vi "Write GIF File (Animated)__ogtk.vi"(6 "delay (ms)":u32[](array[numeric]), 7 "overwrite? (false)":bool, 8 "error in (no error)":errorcluster, 10 "images data":T1[](array[typedef]), 11 "path to GIF file":path) -> (0 "error out":errorcluster, 3 "path":path)   [LabVIEW 2009]
doc: "Writes a multi-frame (animated) Compuserve GIF file. If no path is specified, a file dialog is used to find the file."
uses:
  <vilib>/picture/picture.llb/imagedata.ctl
panel:
  # "Write GIF File (Animated).vi\n\nWrites a multi-frame (animated) Compuserve GIF file. If no path is specified, a file dialog is used to find the file.\n\nPlease visit http://www.OpenG.org to learn about the\nOpen Source LabVIEW software movement.\n\nNOTICE -- YOU MUST LEAVE THIS NOTICE IN PLACE.  PER THE TERMS OF THE LICENSE BELOW, YOU MAY SUBLICENSE THIS SOFTWARE \nIN ANY WAY THAT DOES NOT CONFLICT WITH THIS LICENSE.\n\n### BSD License (http://www.opensource.org/licenses/bsd-license.php) Begin ###\n \nCopyright (c) 2007, Bill Clench <bclench@yahoo.com>\n\nAll rights reserved.\n\nRedistribution and use in source and binary forms, with or without modification, are permitted provided that the following conditions are met:\n\n    * Redistributions of source code must retain the above copyright notice, this list of conditions and the following disclaimer.\n    * Redistributions in binary form must reproduce the above copyright notice, this list of conditions and the following disclaimer in the \n       documentation and/or other materials provided with the distribution.\n    * Neither the name of SciWare, James Kring, Inc., nor the names of its contributors may be used to endorse or promote products derived \n       from this software without specific prior written permission.\n\nTHIS SOFTWARE IS PROVIDED BY THE COPYRIGHT HOLDERS AND CONTRIBUTORS \"AS IS\" AND ANY EXPRESS OR IMPLIED WARRANTIES, \nINCLUDING, BUT NOT LIMITED TO, THE IMPLIED WARRANTIES OF MERCHANTABILITY AND FITNESS FOR A PARTICULAR PURPOSE ARE \nDISCLAIMED. IN NO EVENT SHALL THE COPYRIGHT OWNER OR CONTRIBUTORS BE LIABLE FOR ANY DIRECT, INDIRECT, INCIDENTAL,\n SPECIAL, EXEMPLARY, OR CONSEQUENTIAL DAMAGES (INCLUDING, BUT NOT LIMITED TO, PROCUREMENT OF SUBSTITUTE GOODS OR \nSERVICES; LOSS OF USE, DATA, OR PROFITS; OR BUSINESS INTERRUPTION) HOWEVER CAUSED AND ON ANY THEORY OF LIABILITY, \nWHETHER IN CONTRACT, STRICT LIABILITY, OR TORT (INCLUDING NEGLIGENCE OR OTHERWISE) ARISING IN ANY WAY OUT OF THE USE \nOF THIS SOFTWARE, EVEN IF ADVISED OF THE POSSIBILITY OF SUCH DAMAGE.\n\n### BSD License End ###"
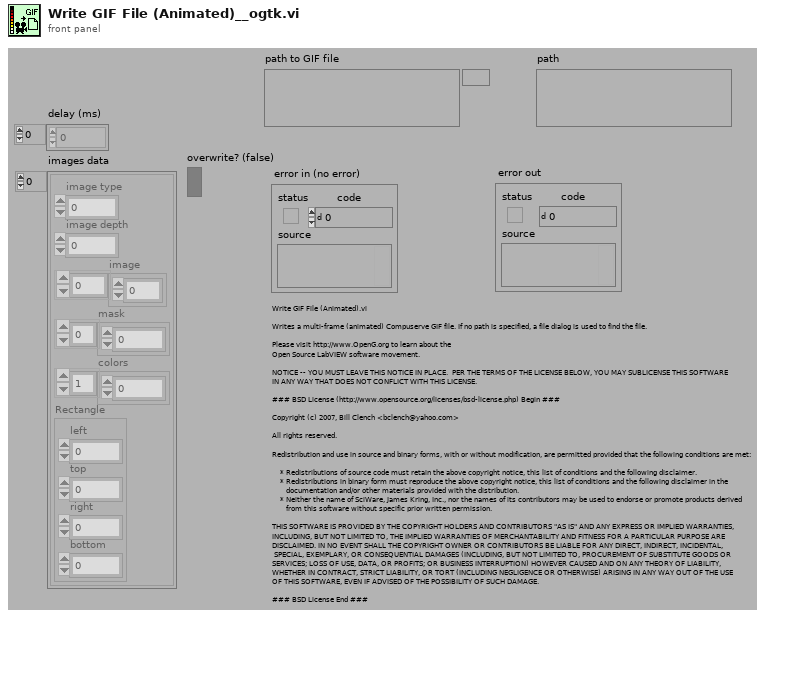
[diagram p1: front panel]
types:
  T1 = typedef "imagedata.ctl" = cluster{"image type":i32, "image depth":i32, "image":u8[], "mask":u8[], "colors":u32[], "Rectangle":cluster{"left":i16, "top":i16, "right":i16, "bottom":i16}}
  T2 = enum32{"existing file", "new file", "new or existing file", "existing dir", "new dir", "new or existing dir", "existing file (use LLBs)", "new file (use LLBs)", "new or existing file (use LLBs)", "new or existing file or directory (use LLBs)", "existing dir (use LLBs)", "new dir (use LLBs)", "new or existing dir (use LLBs)", "existing file or dir", "new file or dir", "new or existing file or dir", "existing file or dir (use LLBs)", "new file or dir (use LLBs)"}
  T3 = enum16{"open", "replace", "create", "open or create", "replace or create", "replace or create with confirmation"}
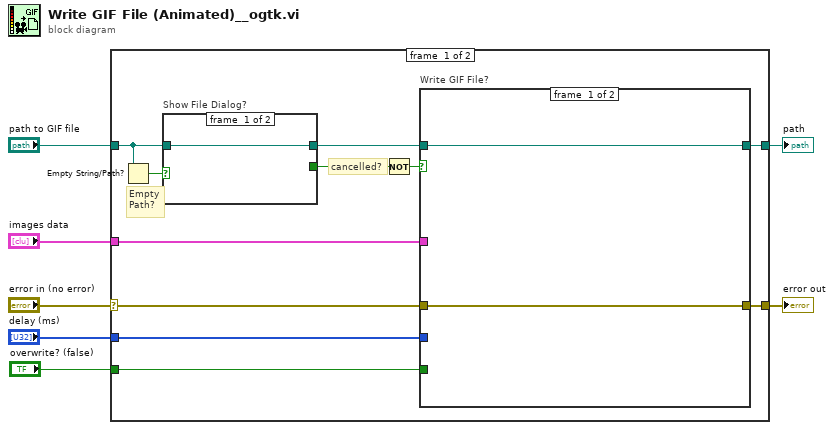
[diagram p0: block diagram]
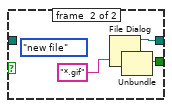
[diagram p2: hidden frame]
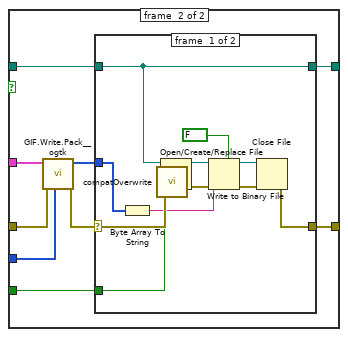
[diagram p3: hidden frame]
diagram:
  n1 = case shown="No Error" "error in (no error)" {
    selector: "error in (no error)" -> [w8 w49]
    tunnel: "images data" -> [w18 _]
    tunnel: [w17 w49] -> w6
    tunnel: "path to GIF file" -> [w15 w50]
    tunnel: "delay (ms)" -> [w12 _]
    tunnel: "overwrite? (false)" -> [w11 _]
    tunnel: [w10 w50] -> w2
    frame #0 {
      # "Empty\nPath?"
      # "cancelled?"
      n2 = Empty String/Path?(string/path=w15) -> (empty?=w16:bool)
      n3 = case "Show File Dialog?" shown="True" w16 {
        tunnel: w15 -> [w19 _]
        tunnel: [w19 w23] -> w13
        tunnel: [_ w21] -> w14
        frame #0 {
        }
        frame #1 {
          (unwired) T2."new file" ("select mode (2)")
          n4 = File Dialog(6:"*.gif") -> (0:w20:errorcluster, 1:w21:bool, 3:w23:path)  [unwired: 6 in, 1 out]
          n5 = Unbundle(w20) -> ()  [unwired: 3 out]
        }
      }
      n6 = Not(x=w14) -> (.not. x?=w9:bool)
      n7 = case "Write GIF File?" shown="True" w9 {
        tunnel: w8 -> [w25 w34]
        tunnel: w18 -> [_ w27]
        tunnel: [w25 w32] -> w17
        tunnel: w13 -> [w24 w30]
        tunnel: w12 -> [_ w29]
        tunnel: w11 -> [_ w28]
        tunnel: [w24 w26] -> w10
        frame #0 {
        }
        frame #1 {
          n8 = call "GIF.Write.Pack__ogtk.vi"("Delay (ms)"=w29, "error in (no error)"=w34, "Images"=w27) -> ("error out"=w33:errorcluster, "Array"=w31:u8[])  [unwired: 7 in]
          n9 = case shown="No Error" w33 {
            selector: w33 -> [w46 w48]
            tunnel: [w45 w48] -> w32
            tunnel: w31 -> [w44 _]
            tunnel: w30 -> [w41 w47]
            tunnel: w28 -> [w42 _]
            tunnel: [w41 w47] -> w26
            frame #0 {
              n10 = Byte Array To String(unsigned byte array=w44) -> (string=w43:string)
              n11 = call <vilib>:"compatOverwrite.vi"("overwrite (F)"=w42) -> ("overwrite?"=w35:T3)
              n12 = Open/Create/Replace File(file path (use dialog)=w41, error in=w46, operation (0:open)=w35) -> (refnum out=w40:refnum<file>, error out=w39:errorcluster)  [unwired: 3 in, 1 out]
              n13 = Write to Binary File(file (use dialog)=w40, data=w43, error in=w39, 5:FALSE ("prepend array or string size? (T)")) -> (refnum out=w38:refnum<file>, error out=w37:errorcluster)  [unwired: 2 in, 1 out]
              n14 = Close File(refnum=w38, error in=w37) -> (error out=w45:errorcluster)  [unwired: 1 out]
            }
            frame #1 {
            }
          }
        }
      }
    }
    frame #1 {
    }
  }
  "error out" <- w6
  "path" <- w2
